vi "ReadLockinData_ETH.vi"(2 "error in":T1, 3 "Lockin Address":string="0:8") -> (0 "error out":T1, 1 "Complex measurement values":cdb[](array[numeric]))   [LabVIEW 2023]
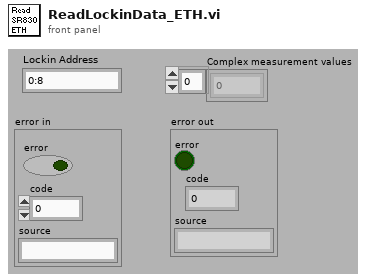
[diagram p1: front panel]
types:
  T1 = cluster{"error":bool, "code":i32, "source":string}
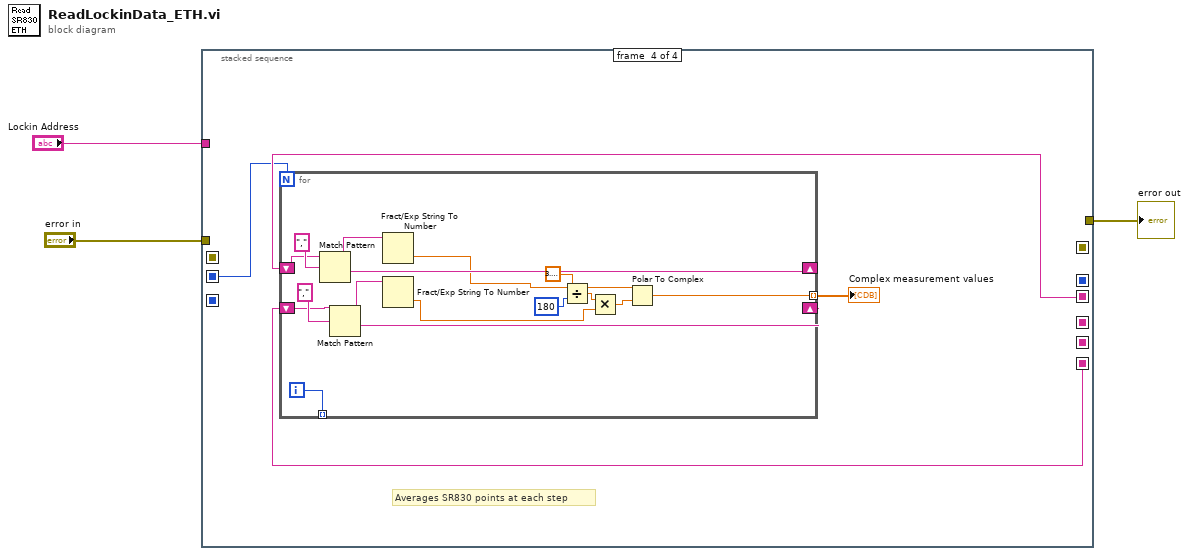
[diagram p0: block diagram]
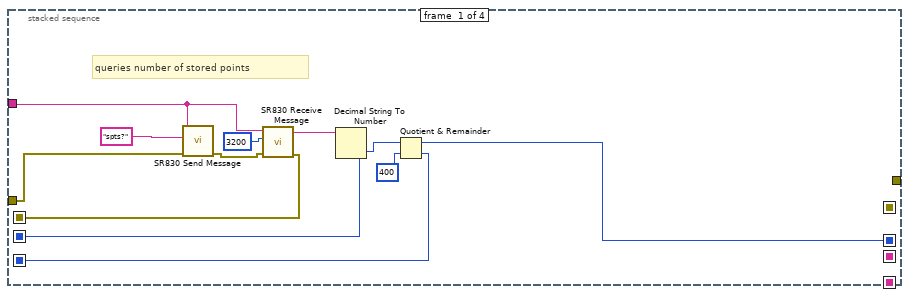
[diagram p2: hidden frame]
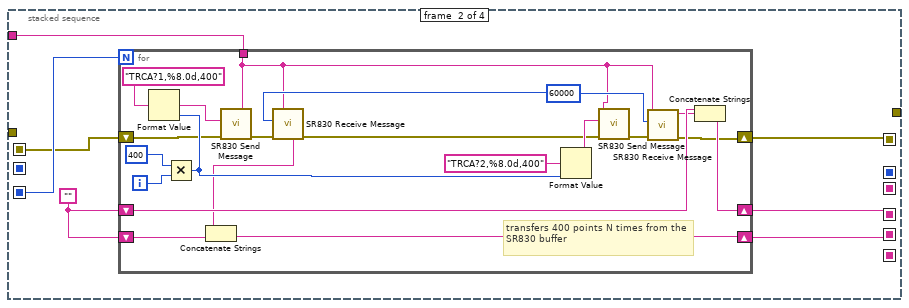
[diagram p3: hidden frame]
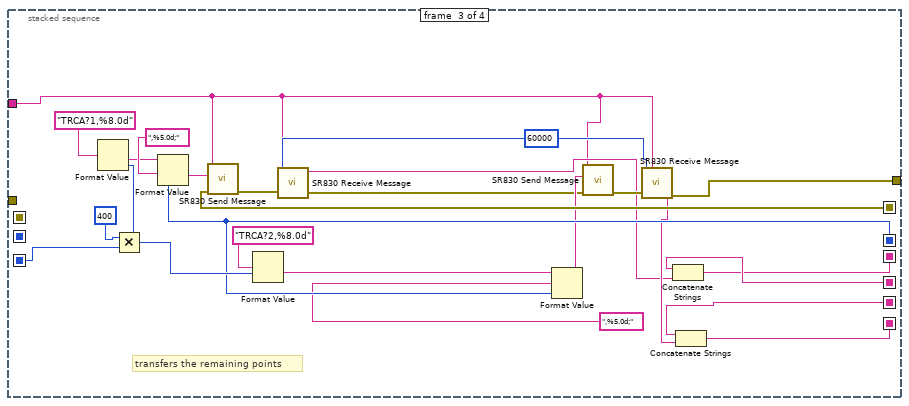
[diagram p4: hidden frame]
diagram:
  n1 = stacked-sequence {
    seq-local: [w8 _ _ _] -> [_ _ w64 _]
    seq-local: [_ w20 _ _] -> [_ _ w61 _]
    seq-local: [_ w19 _ _] -> [_ _ w63 _]
    seq-local: [_ w18 _ _] -> [_ _ w62 _]
    seq-local: [_ _ w46 _] -> [_ _ _ w69]
    seq-local: [_ _ w45 _] -> [_ _ _ w70]
    seq-local: [w9 _ _ _] -> [_ _ _ w68]
    seq-local: [w7 _ _ _] -> [_ w16 w42 _]
    seq-local: [w4 _ _ _] -> [_ w15 _ _]
    tunnel: [_ _ w44 _] -> w1
    tunnel: "Lockin Address" -> [w13 w17 w43 _]
    tunnel: "error in" -> [w6 _ _ _]
    frame #0 {
      # "queries number of stored points"
      n2 = call "SR830 Send Message.vi"("address string"=w13, "write buffer"="spts?", "error in"=w6) -> ("error out"=w5:T1)  [unwired: 4 in, 2 out]
      n3 = call "SR830 Receive Message.vi"("address string"=w13, "byte count"=3200, "error in"=w5) -> ("read buffer"=w11:string, "error out"=w4:T1)  [unwired: 4 in, 1 out]
      n4 = Decimal String To Number(string=w11) -> (number=w9:i32)  [unwired: 2 in, 1 out]
      n5 = Quotient & Remainder(x=w9, y=400) -> (x-y*floor(x/y)=w8:i32, floor(x/y)=w7:i32)
    }
    frame #1 {
      w21 = ""
      n6 = for {
        N: w16 -> [_]
        shift-right: [w27] -> w20
        shift-left: w15 -> [w34]
        shift-right: [w39] -> w18
        shift-left: w21 -> [w38]
        shift-right: [w35] -> w19
        shift-left: w21 -> [w36]
        tunnel: w17 -> [w22]
        i -> [w41]
        w28 = 60000
        # "transfers 400 points N times from the SR830 buffer"
        n7 = Multiply(x=400, y=w41) -> (x*y=w37:i32)
        n8 = Format Value(format string="TRCA?1,%8.0d,400", value (0)=w37) -> (output string=w32:string)  [unwired: 1 in]
        n9 = call "SR830 Send Message.vi"("address string"=w22, "write buffer"=w32, "error in"=w34) -> ("error out"=w33:T1)  [unwired: 4 in, 2 out]
        n10 = call "SR830 Receive Message.vi"("address string"=w22, "byte count"=w28, "error in"=w33) -> ("read buffer"=w31:string, "error out"=w29:T1)  [unwired: 4 in, 1 out]
        n11 = Concatenate Strings(w31, w38) -> (w39:string)
        n12 = Format Value(format string="TRCA?2,%8.0d,400", value (0)=w37) -> (output string=w30:string)  [unwired: 1 in]
        n13 = call "SR830 Send Message.vi"("address string"=w22, "write buffer"=w30, "error in"=w29) -> ("error out"=w26:T1)  [unwired: 4 in, 2 out]
        n14 = call "SR830 Receive Message.vi"("address string"=w22, "byte count"=w28, "error in"=w26) -> ("read buffer"=w25:string, "error out"=w27:T1)  [unwired: 4 in, 1 out]
        n15 = Concatenate Strings(w36, w25) -> (w35:string)
      }
    }
    frame #2 {
      w55 = 60000
      # "transfers the remaining points"
      n16 = Multiply(x=400, y=w42) -> (x*y=w65:i32)
      n17 = Format Value(format string="TRCA?1,%8.0d", value (0)=w65) -> (output string=w51:string)  [unwired: 1 in]
      n18 = Format Value(string ("")=w51, format string=",%5.0d;", value (0)=w64) -> (output string=w50:string)
      n19 = call "SR830 Send Message.vi"("address string"=w43, "write buffer"=w50, "error in"=w61) -> ("error out"=w57:T1)  [unwired: 4 in, 2 out]
      n20 = Format Value(format string="TRCA?2,%8.0d", value (0)=w65) -> (output string=w47:string)  [unwired: 1 in]
      n21 = call "SR830 Receive Message.vi"("address string"=w43, "byte count"=w55, "error in"=w57) -> ("read buffer"=w56:string, "error out"=w54:T1)  [unwired: 4 in, 1 out]
      n22 = Format Value(string ("")=w47, format string=",%5.0d;", value (0)=w64) -> (output string=w60:string)
      n23 = call "SR830 Send Message.vi"("address string"=w43, "write buffer"=w60, "error in"=w54) -> ("error out"=w59:T1)  [unwired: 4 in, 2 out]
      n24 = call "SR830 Receive Message.vi"("address string"=w43, "byte count"=w55, "error in"=w59) -> ("read buffer"=w58:string, "error out"=w44:T1)  [unwired: 4 in, 1 out]
      n25 = Concatenate Strings(w63, w56) -> (w46:string)
      n26 = Concatenate Strings(w62, w58) -> (w45:string)
    }
    frame #3 {
      # "Averages SR830 points at each step"
      n27 = for {
        N: w68 -> [_]
        shift-right: [w82] -> _
        shift-left: w69 -> [w81]
        shift-right: [w80] -> _
        shift-left: w70 -> [w79]
        tunnel: [w78] -> _ mode=indexing
        tunnel: [w71] -> w67 mode=indexing
        i -> [w78]
        n28 = Match Pattern(string=w81, regular expression=",") -> (before substring=w85:string, after substring=w82:string)  [unwired: 1 in, 2 out]
        n29 = Match Pattern(string=w79, regular expression=",") -> (before substring=w84:string, after substring=w80:string)  [unwired: 1 in, 2 out]
        n30 = Fract/Exp String To Number(string=w85) -> (number=w73:dbl)  [unwired: 3 in, 1 out]
        n31 = Fract/Exp String To Number(string=w84) -> (number=w77:dbl)  [unwired: 3 in, 1 out]
        n32 = Divide(x=3.141592653589793, y=180) -> (x/y=w74:dbl)
        n33 = Multiply(x=w74, y=w77) -> (x*y=w72:dbl)
        n34 = Polar To Complex(1:w72, 2:w73) -> (0:w71:cdb)
      }
      "Complex measurement values" <- w67
    }
  }
  "error out" <- w1
